vi "RDS Msg To String.vi"(8 "error in (no error)":errorcluster, 11 "RDS Message in":refnum<class "RDS Message.lvclass">) -> (0 "error out":errorcluster, 2 "String":string, 3 "RDS Message out":refnum<class "RDS Message.lvclass">)   [LabVIEW 2015, in "RDS Child Messages.lvlib" / "RDS Message.lvclass"]
uses:
  RDS Message.lvclass
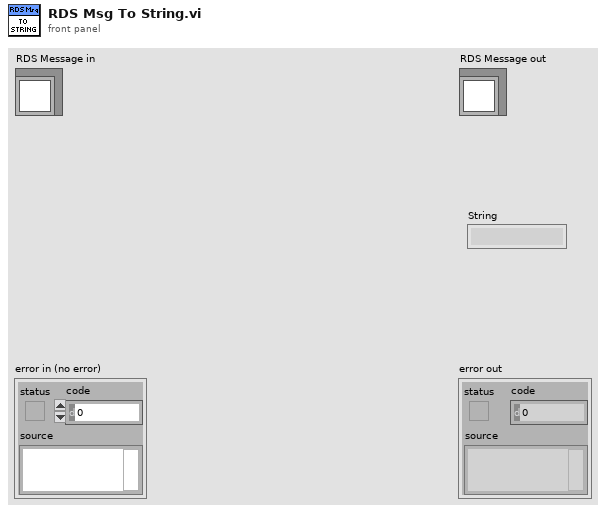
[diagram p1: front panel]
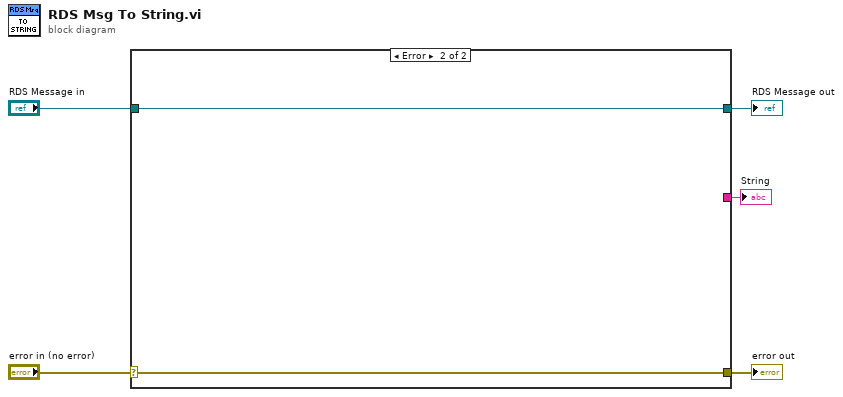
[diagram p0: block diagram]
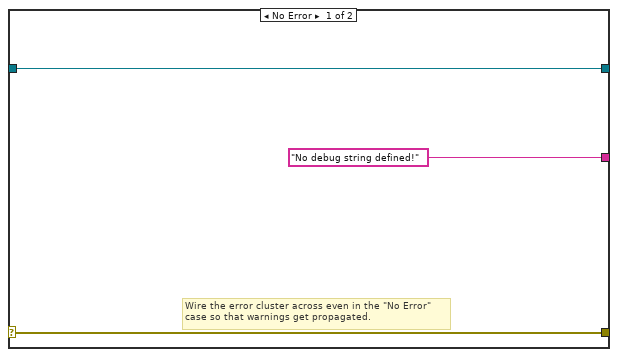
[diagram p2: hidden frame]
diagram:
  n1 = case shown="Error" "error in (no error)" {
    selector: "error in (no error)" -> [w7 w10]
    tunnel: [w7 w10] -> w4
    tunnel: [w8 w9] -> w2
    tunnel: "RDS Message in" -> [w8 w9]
    tunnel: ["No debug string defined!" _] -> w1
    frame No Error {
      # "Wire the error cluster across even in the \"No Error\"\ncase so that warnings get propagated."
    }
    frame Error {
    }
  }
  "error out" <- w4
  "RDS Message out" <- w2
  "String" <- w1
